vi "RELAYS Write the Baudrate.vi"(8 "error in (no error)":errorcluster, 9 "baudrate":T1=3 items=["4800"=2, "9600"=3, "19200"=4], 10 "Dev addr":u8=1 format="%x", 11 "VISA resource name":refnum<visa-resource-name>) -> (0 "error out":errorcluster, 1 "success?":bool, 2 "ack":string, 3 "VISA resource name out":refnum<visa-resource-name>)   [LabVIEW 2016, in "MB _relays.lvlib"]
uses:
  MB _relays.lvlib
  type defs/baudrate.ctl
  private/gen MB frame -Set the Baudrate.vi
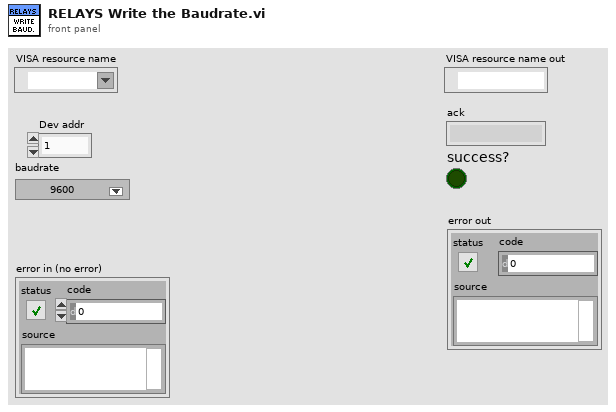
[diagram p1: front panel]
types:
  T1 = typedef "MB _relays.lvlib/baudrate.ctl" = u8
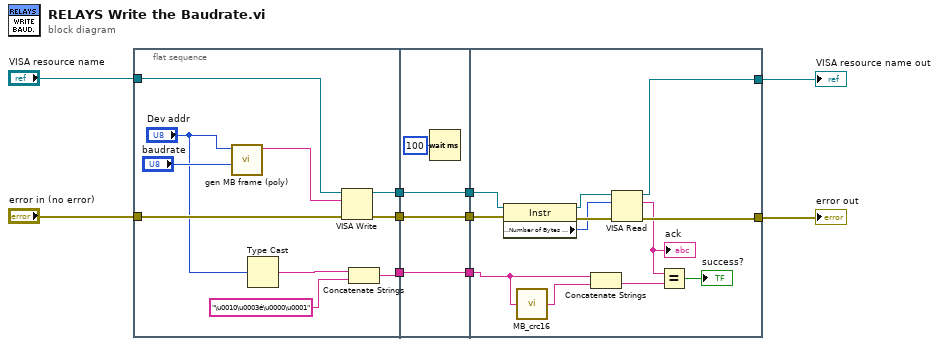
[diagram p0: block diagram]
diagram:
  n1 = flat-sequence {
    tunnel: "error in (no error)" -> [w17]
    tunnel: "VISA resource name" -> [w16]
    tunnel: [w20] -> w6
    tunnel: [w19] -> w5
    tunnel: [w11] -> w1
    tunnel: w6 -> [w24]
    tunnel: w5 -> [w23]
    tunnel: [w24] -> w4
    tunnel: [w23] -> w3
    tunnel: [w21] -> w2
    tunnel: w1 -> [w21]
    tunnel: [w30] -> w9
    tunnel: [w31] -> w10
    tunnel: w4 -> [w35]
    tunnel: w3 -> [w36]
    tunnel: w2 -> [w29]
    frame #0 {
      n2 = call-poly "gen MB frame (poly).vi"("baudrate"="baudrate", "Dev Addr"="Dev addr") -> ("MB frame"=w18:string)  [unwired: 9 in]
      n3 = Type Cast(x="Dev addr") -> (*(type *) &x=w12:string)  [unwired: 1 in]
      n4 = VISA Write(VISA resource name=w16, write buffer=w18, error in (no error)=w17) -> (VISA resource name out=w20:refnum<visa-resource-name>, error out=w19:errorcluster)  [unwired: 1 out]
      n5 = Concatenate Strings(w12, "\u0010\u0003é\u0000\u0001") -> (w11:string)
    }
    frame #1 {
      n6 = Wait (ms)(milliseconds to wait=u32 100) -> ()  [unwired: 1 out]
    }
    frame #2 {
      n7 = property class="Instr"(reference=w35, error in=w36) -> (reference out=w33:refnum<visa-resource-name>, error out=w34:errorcluster, "Serial Settings:Number of Bytes at Serial Port"=w32:u32)
      n8 = call "MB_crc16.vi"("message"=w29) -> ("CRC16"=w28:string)  [unwired: 4 in]
      n9 = Concatenate Strings(w29, w28) -> (w27:string)
      n10 = VISA Read(VISA resource name=w33, byte count=w32, error in (no error)=w34) -> (VISA resource name out=w31:refnum<visa-resource-name>, read buffer=w26:string, error out=w30:errorcluster)  [unwired: 1 out]
      "ack" <- w26
      n11 = Equal?(x=w26, y=w27) -> (x = y?=→"success?":bool)
    }
  }
  "VISA resource name out" <- w10
  "error out" <- w9
